vi "ScreenShotFrontPannel.vi"(8 "error in (no error)":errorcluster, 9 "SubFolderName":string, 10 "FileName":string="Test", 11 "vi path":path) -> (0 "error out":errorcluster)   [LabVIEW 2020]
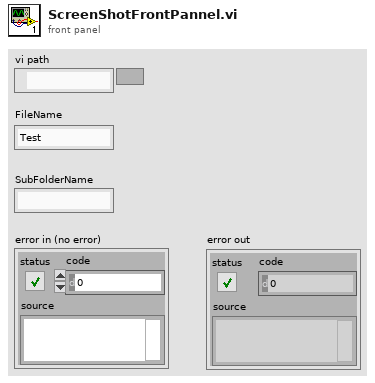
[diagram p1: front panel]
types:
  T1 = typedef "imagedata.ctl" = cluster{"image type":i32, "image depth":i32, "image":u8[], "mask":u8[], "colors":u32[], "Rectangle":cluster{"left":i16, "top":i16, "right":i16, "bottom":i16}}
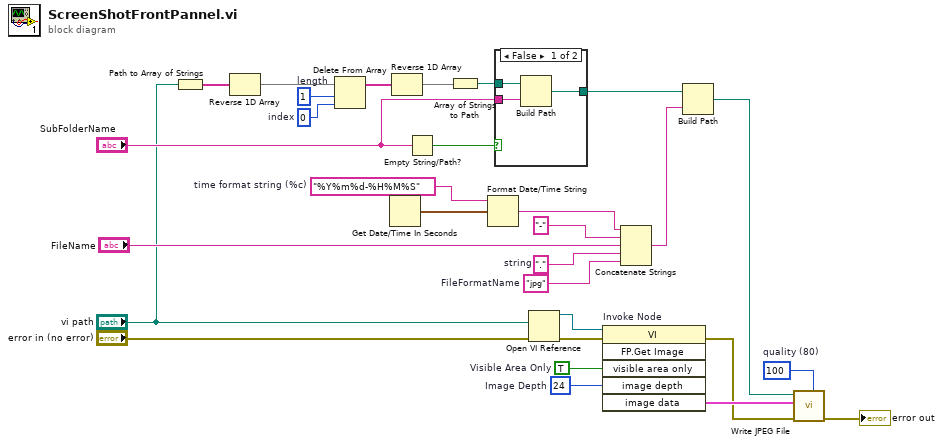
[diagram p0: block diagram]
diagram:
  w4 = 1  # length
  w5 = 0  # index
  w13 = "jpg"  # FileFormatName
  w15 = "."  # string
  w19 = "%Y%m%d-%H%M%S"  # time format string (%c)
  w22 = 24  # Image Depth
  w23 = 100  # quality (80)
  w27 = TRUE  # Visible Area Only
  n1 = Path to Array of Strings(0:"vi path") -> (2:w7:string[])  [unwired: 1 out]
  n2 = Reverse 1D Array(array=w7) -> (reversed array=w6:string[])
  n3 = Delete From Array "Delete From Array"(array=w6, length=w4, index=w5) -> (array with subset deleted=w3:string[])  [unwired: 1 out]
  n4 = Get Date/Time In Seconds() -> (seconds since 1Jan1904=w20:timestamp)
  n5 = Reverse 1D Array(array=w3) -> (reversed array=w2:string[])
  n6 = Empty String/Path?(string/path="SubFolderName") -> (empty?=w11:bool)
  n7 = Array of Strings to Path(0:w2) -> (2:w1:path)  [unwired: 1 in]
  n8 = Format Date/Time String(time format string (%c)=w19, seconds (now)=w20) -> (date/time string=w14:string)  [unwired: 1 in]
  n9 = case shown="False" w11 {
    tunnel: w1 -> [w32 w33]
    tunnel: [w31 w33] -> w12
    tunnel: "SubFolderName" -> [w30 _]
    frame False {
      n10 = Build Path(base path=w32, name or relative path=w30) -> (appended path=w31:path)
    }
    frame True {
    }
  }
  n11 = Open VI Reference(vi path="vi path", error in (no error)="error in (no error)") -> (vi reference=w29:refnum<vi>, error out=w28:errorcluster)  [unwired: 4 in]
  n12 = invoke on="Invoke Node" class="VI" method="FP.Get Image"(reference=w29, error in=w28, "visible area only"=w27, "image depth"=w22) -> (error out=w25:errorcluster, "image data"=w26:T1)  [unwired: 2 in, 4 out]
  n13 = Concatenate Strings "Concatenate Strings"(w14, "-", "FileName", w15, w13) -> (w18:string)
  n14 = Build Path(base path=w12, name or relative path=w18) -> (appended path=w9:path)
  n15 = call <vilib>:"Write JPEG File.vi"("quality (80)"=w23, "error in (no error)"=w25, "image data"=w26, "path to JPEG file"=w9) -> ("error out"=→"error out":errorcluster)  [unwired: 6 in, 1 out]
